vi "Version Maker - backup.vi"(5 "File name (including .ini)":path, 6 "Section":string="Simulator", 7 "Folder Path containing version information":path, 8 "Error In":errorcluster, 9 "This VI ref":refnum<vi>, 10 "Open Application Reference":refnum<vi>, 11 "Current VI's Path":path) -> (0 "Error Out":errorcluster)   [LabVIEW 2014]
doc: "It is part of HIL Change Management System. \n\nThis VI sets the front panel title, keeps track of the versions of the executable, and registers the executable version in a file that can be used for updating the change registry.\n\nSee the help."
uses:
  <vilib>/Utility/config.llb/Read Key (Boolean).vi
  <vilib>/Utility/config.llb/Write Key (String).vi
  <vilib>/Utility/config.llb/Write Key (Boolean).vi
  <vilib>/Utility/config.llb/Read Key (String).vi
  <vilib>/Utility/config.llb/NI_LVConfig.lvlib
  <vilib>/Utility/file.llb/Write To Spreadsheet File (string).vi
panel:
  out "appended path":path
  # "Change Management System - Version Control"
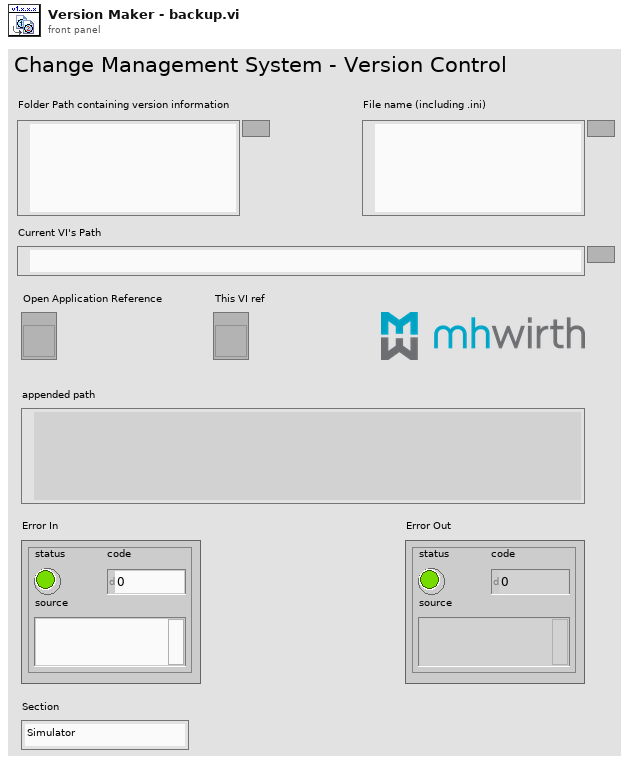
[diagram p1: front panel]
types:
  T1 = typedef "NI_LVConfig.lvlib/Config Data RefNum.ctl" = refnum<k1>
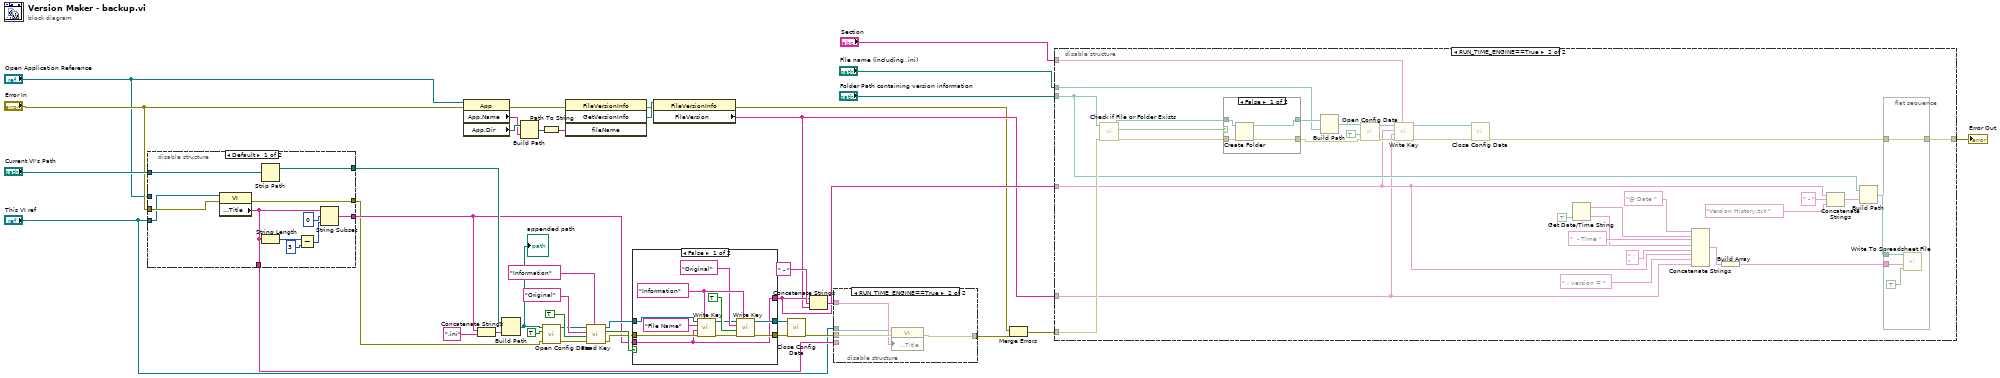
[diagram p0: block diagram]
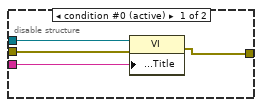
[diagram p4: hidden frame]
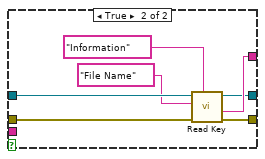
[diagram p5: hidden frame]
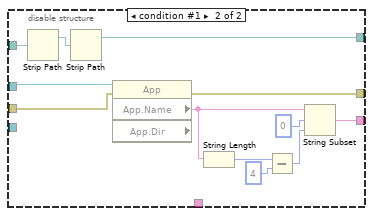
[diagram p6: hidden frame]
diagram:
  n1 = disable-structure shown="Default" {
    disable-tunnel: "Current VI's Path" -> [w44 w64]
    disable-tunnel: [w52 w62] -> w40
    disable-tunnel: [w47 w56] -> w20
    disable-tunnel: "Error In" -> [w43 w54]
    disable-tunnel: "Open Application Reference" -> [_ w55]
    disable-tunnel: [w46 w53] -> w10
    disable-tunnel: [w45 _] -> w9
    disable-tunnel: "This VI ref" -> [w42 _]
    frame condition #0 (active) {
      n2 = property class="VI"(reference=w42, error in=w43) -> (error out=w46:errorcluster, "Front Panel.Title"=w45:string)  [unwired: 1 out]
      n3 = Strip Path(path=w44) -> (stripped path=w52:path)  [unwired: 1 out]
      n4 = String Length(string=w45) -> (length=w49:i32)
      n5 = Subtract(x=w49, y=3) -> (x-y=w51:i32)
      n6 = String Subset(string=w45, offset (0)=0, length (rest)=w51) -> (substring=w47:string)
    }
    frame condition #1 {
      n7 = Strip Path(path=w64) -> (stripped path=w63:path)  [unwired: 1 out]
      n8 = Strip Path(path=w63) -> (stripped path=w62:path)  [unwired: 1 out]
      n9 = property class="App" props=["App.Name", "App.Dir"](reference=w55, error in=w54) -> (error out=w53:errorcluster, "App.Name"=w57:string)  [unwired: 2 out]
      n10 = String Length(string=w57) -> (length=w59:i32)
      n11 = Subtract(x=w59, y=4) -> (x-y=w61:i32)
      n12 = String Subset(string=w57, offset (0)=0, length (rest)=w61) -> (substring=w56:string)
    }
  }
  n13 = property class="App"(reference="Open Application Reference", error in="Error In") -> (error out=w17:errorcluster, "App.Name"=w25:string, "App.Dir"=w26:path)  [unwired: 1 out]
  n14 = Concatenate Strings(w20, ".ini" ("string")) -> (w22:string)
  n15 = Build Path(base path=w40, name or relative path=w22) -> (appended path=w39:path)
  "appended path" <- w39
  n16 = Build Path(base path=w26, name or relative path=w25) -> (appended path=w27:path)
  n17 = Path To String(path=w27) -> (string=w24:string)
  n18 = call <vilib>:"Open Config Data.vi"("error in (no error)"=w10, "create file if necessary (T)"=TRUE, "configuration file path"=w39) -> ("error out"=w18:errorcluster, "refnum"=w19:T1)  [unwired: 6 in, 1 out]
  n19 = invoke class="FileVersionInfo" method="GetVersionInfo"(error in=w17, "fileName"=w24) -> (error out=w16:errorcluster, "GetVersionInfo"=w28:refnum<k24>)  [unwired: 2 in, 2 out]
  n20 = call-poly <vilib>:"Read Key.vi"("section"="Information", "error in (no error)"=w18, "default value"=TRUE ("create file if necessary (T)"), "key"="Original", "refnum"=w19) -> ("error out"=w34:errorcluster, "found?"=w35:bool, "refnum out"=w33:T1)  [unwired: 3 in, 1 out]
  n21 = case shown="False" w35 {
    tunnel: w34 -> [w75 w81]
    tunnel: w33 -> [w74 w82]
    tunnel: [w67 w79] -> w32
    tunnel: [w66 w78] -> w31
    tunnel: w20 -> [w65 _]
    tunnel: [w65 w80] -> w15
    frame False {
      w72 = "Information" ("section")
      n22 = call-poly <vilib>:"Write Key.vi"("section"=w72, "error in (no error)"=w75, "value"=w65, "key"="File Name", "refnum"=w74) -> ("error out"=w69:errorcluster, "refnum out"=w68:T1)  [unwired: 4 in, 1 out]
      n23 = call-poly <vilib>:"Write Key.vi"("section"=w72, "error in (no error)"=w69, "value"=TRUE ("create file if necessary (T)"), "key"="Original", "refnum"=w68) -> ("error out"=w66:errorcluster, "refnum out"=w67:T1)  [unwired: 4 in, 1 out]
    }
    frame True {
      n24 = call-poly <vilib>:"Read Key.vi"("section"="Information", "error in (no error)"=w81, "key"="File Name", "refnum"=w82) -> ("error out"=w78:errorcluster, "value"=w80:string, "refnum out"=w79:T1)  [unwired: 4 in, 1 out]
    }
  }
  n25 = property class="FileVersionInfo"(reference=w28, error in=w16) -> (error out=w6:errorcluster, "FileVersion"=w14:string)  [unwired: 1 out]
  n26 = call <vilib>:"Close Config Data.vi"("error in (no error)"=w31, "refnum"=w32) -> ("error out"=w30:errorcluster)  [unwired: 8 in, 1 out]
  n27 = Concatenate Strings(w15, " - " ("section"), w14) -> (w23:string)
  n28 = disable-structure shown="RUN_TIME_ENGINE==True" {
    disable-tunnel: w30 -> [w86 w90]
    disable-tunnel: w23 -> [_ w89]
    disable-tunnel: [w84 w88] -> w7
    disable-tunnel: w9 -> [w85 _]
    disable-tunnel: "This VI ref" -> [w83 w87]
    frame condition #0 (active) {
      n29 = property class="VI"(reference=w83, error in=w86, "Front Panel.Title"=w85) -> (error out=w84:errorcluster)  [unwired: 1 out]
    }
    frame condition #1 {
      n30 = property class="VI"(reference=w87, error in=w90, "Front Panel.Title"=w89) -> (error out=w88:errorcluster)  [unwired: 1 out]
    }
  }
  n31 = Merge Errors(w6, w7) -> (w3:errorcluster)
  n32 = disable-structure shown="RUN_TIME_ENGINE==True" {
    disable-tunnel: w15 -> [_ w93]
    disable-tunnel: w14 -> [_ w92]
    disable-tunnel: w3 -> [w91 w98]
    disable-tunnel: "File name (including .ini)" -> [_ w99]
    disable-tunnel: "Folder Path containing version information" -> [_ w97]
    disable-tunnel: [w91 w95] -> w2
    disable-tunnel: "Section" -> [_ w94]
    frame condition #0 (active) {
    }
    frame condition #1 {
      n33 = call <vilib>:"Check if File or Folder Exists.vi"("error in (no error)"=w98, "path"=w97) -> ("error out"=w107:errorcluster, "file or folder exists?"=w108:bool, "dup path"=w109:path)  [unwired: 7 in]
      n34 = case shown="False" w108 {
        tunnel: [w127 w129] -> w101
        tunnel: w109 -> [w126 w129]
        tunnel: w107 -> [w125 w128]
        tunnel: [w124 w128] -> w100
        frame False {
          n35 = Create Folder(path (use dialog)=w126, error in=w125) -> (created path=w127:path, error out=w124:errorcluster)  [unwired: 1 in, 1 out]
        }
        frame True {
        }
      }
      n36 = Build Path(base path=w101, name or relative path=w99) -> (appended path=w105:path)
      n37 = call <vilib>:"Open Config Data.vi"("error in (no error)"=w100, "create file if necessary (T)"=TRUE, "configuration file path"=w105) -> ("error out"=w110:errorcluster, "refnum"=w104:T1)  [unwired: 6 in, 1 out]
      n38 = call-poly <vilib>:"Write Key.vi"("section"=w94, "error in (no error)"=w110, "value"=w92, "key"=w93, "refnum"=w104) -> ("error out"=w102:errorcluster, "refnum out"=w103:T1)  [unwired: 4 in, 1 out]
      n39 = call <vilib>:"Close Config Data.vi"("error in (no error)"=w102, "refnum"=w103) -> ("error out"=w96:errorcluster)  [unwired: 8 in, 1 out]
      n40 = Get Date/Time String(want seconds? (F)=TRUE) -> (date string=w115:string, time string=w113:string)  [unwired: 2 in]
      n41 = Concatenate Strings("@ Date " ("section"), w115, "  - Time " ("section"), w113, " ; " ("section"), w93, " ; version = " ("section"), w92) -> (w119:string)
      n42 = Build Array(w119) -> (w118:string[])
      n43 = Concatenate Strings(w93, " - " ("section"), "Version History.txt " ("section")) -> (w123:string)
      n44 = Build Path(base path=w97, name or relative path=w123) -> (appended path=w120:path)
      n45 = flat-sequence {
        tunnel: w120 -> [w133]
        tunnel: w118 -> [w131]
        tunnel: [w130] -> w95
        tunnel: w96 -> [w130]
        frame #0 {
          n46 = call-poly <vilib>:"Write To Spreadsheet File.vi"("append to file? (new file:F)"=TRUE, "1D data"=w131, "file path (dialog if empty)"=w133) -> ()  [unwired: 5 in, 1 out]
        }
      }
    }
  }
  "Error Out" <- w2
